vi "rtin_controlRealTimeInChangePerPulse.vi"(7 "Set":bool, 8 "error in":errorcluster, 9 "delta":i32, 10 "axis in":i32, 11 "connection ID":refnum<k5>) -> (0 "error out":errorcluster, 1 "delta":i32, 2 "axis out":i32, 3 "connection ID":refnum<k5>)   [LabVIEW 2016]
doc: "This function retrieves or sets the change per pulse for the selected axis under real time input in the closed-loop mode."
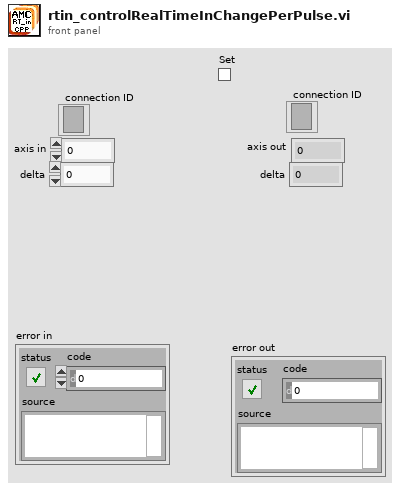
[diagram p1: front panel]
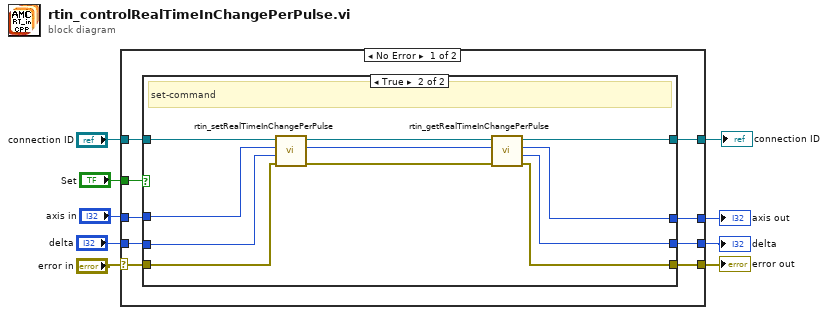
[diagram p0: block diagram]
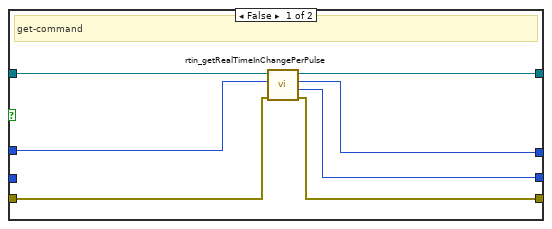
[diagram p2: hidden frame]
diagram:
  n1 = case shown="No Error" "error in" {
    selector: "error in" -> [w14 w40]
    tunnel: "axis in" -> [w18 w37]
    tunnel: [w10 w40] -> w8
    tunnel: "delta" -> [w16 w38]
    tunnel: [w13 w38] -> w3
    tunnel: "Set" -> [w15 _]
    tunnel: [w12 w39] -> w6
    tunnel: "connection ID" -> [w17 w39]
    tunnel: [w11 w37] -> w1
    frame No Error {
      n2 = case shown="True" w15 {
        tunnel: w17 -> [w25 w33]
        tunnel: w18 -> [w21 w30]
        tunnel: w16 -> [_ w28]
        tunnel: w14 -> [w23 w29]
        tunnel: [w20 w26] -> w13
        tunnel: [w24 w32] -> w12
        tunnel: [w19 w31] -> w11
        tunnel: [w22 w27] -> w10
        frame False {
          # "get-command"
          n3 = call "rtin_getRealTimeInChangePerPulse.vi"("error in"=w23, "axis"=w21, "connection ID"=w25) -> ("error out"=w22:errorcluster, "resolution"=w20:i32, "axis_out"=w19:i32, "connection ID"=w24:refnum<k5>)  [unwired: 5 in]
        }
        frame True {
          # "set-command"
          n4 = call "rtin_setRealTimeInChangePerPulse.vi"("error in"=w29, "delta"=w28, "axis"=w30, "connection ID"=w33) -> ("error out"=w34:errorcluster, "axis_out"=w35:i32, "connection ID"=w36:refnum<k5>)  [unwired: 5 in]
          n5 = call "rtin_getRealTimeInChangePerPulse.vi"("error in"=w34, "axis"=w35, "connection ID"=w36) -> ("error out"=w27:errorcluster, "resolution"=w26:i32, "axis_out"=w31:i32, "connection ID"=w32:refnum<k5>)  [unwired: 5 in]
        }
      }
    }
    frame Error {
    }
  }
  "error out" <- w8
  "axis out" <- w1
  "delta" <- w3
  "connection ID" <- w6
